vi "Set RF Power.vi"(8 "error in (no error)":errorcluster, 10 "Step In":refnum<k7>, 11 "Harmonics in":refnum<class "Harmonics.lvclass">) -> (0 "error out":errorcluster, 2 "Step Out":refnum<k7>, 3 "Harmonics out":refnum<class "Harmonics.lvclass">)   [LabVIEW 2018, in "Harmonics.lvlib" / "Harmonics.lvclass"]
uses:
  Harmonics.lvclass
  C:/Sequence Automation/Plugins/Measurement Interface.lvlibp/Measurement Interface.lvclass
  Plugins/Measurement Interface.lvlibp/Private Methods/Measurement Name/Read Measurement Name.vi
  Plugins/TestStand API Tools (TSAT).lvlibp/Step Actions/TSAT Step Actions.lvlib
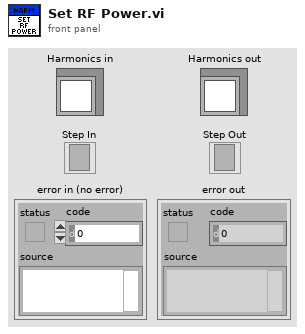
[diagram p1: front panel]
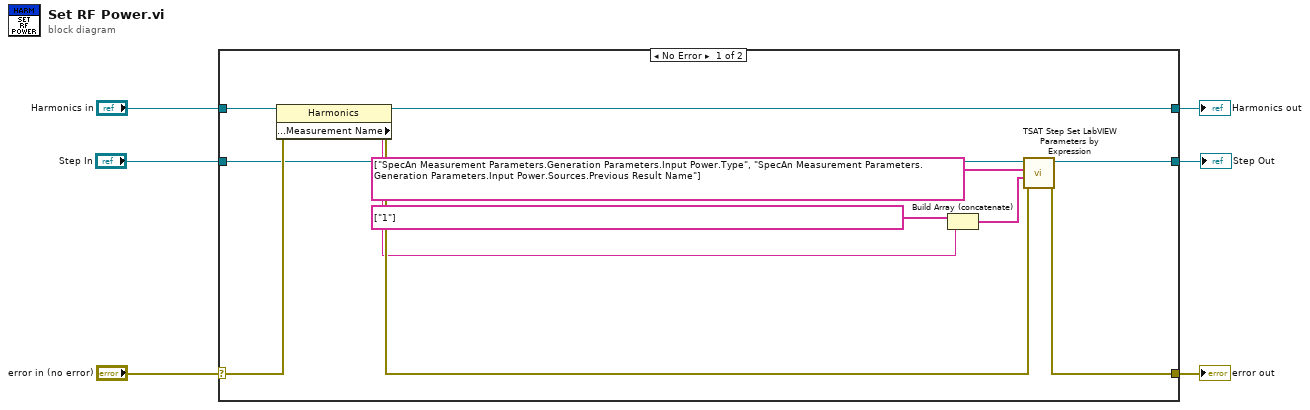
[diagram p0: block diagram]
diagram:
  n1 = case shown="No Error" "error in (no error)" {
    selector: "error in (no error)" -> [w17 w20]
    tunnel: [w11 w20] -> w5
    tunnel: [w15 w19] -> w3
    tunnel: "Harmonics in" -> [w16 w19]
    tunnel: "Step In" -> [w14 w18]
    tunnel: [w13 w18] -> w1
    frame No Error {
      n2 = property class="Harmonics"(reference=w16, error in=w17) -> (reference out=w15:refnum<class "Harmonics.lvclass">, error out=w12:errorcluster, "Public Methods:Measurement Name"=w7:string)
      n3 = Build Array (concatenate)(string[] ["1"] ("Value Expressions"), w7) -> (w8:string[])
      n4 = call "TSAT Step Set LabVIEW Parameters by Expression.vi"("Error In"=w12, "Value Expressions"=w8, "Parameters to Set"=string[] ["SpecAn Measurement Parameters.Generation Parameters.Input Power.Type", "SpecAn Measurement Parameters.Generation Parameters.Input Power.Sources.Previous Result Name"], "Step In"=w14) -> ("Error Out"=w11:errorcluster, "Step Out"=w13:refnum<k7>)  [unwired: 6 in]
    }
    frame Error {
    }
  }
  "error out" <- w5
  "Harmonics out" <- w3
  "Step Out" <- w1
